vi "Periodic Tasks.vi"(8 "error in":errorcluster) -> ()   [LabVIEW 2013]
doc: "This VI runs in parallel to other tasks. It can contain as many user-defined periodic loops as you need. These can carry out PID or other sorts of timed response."
uses:
  <vilib>/Rock Robotics/SystemInterfaces/Utilities/FPGA_UtilitiesLED Source.ctl
  <vilib>/Rock Robotics/SystemInterfaces/Utilities/FPGA_UtilitiesLED State.ctl
  Robot Global Data.vi
  RefnameEnum.ctl
  SingleSolenoidAction.ctl
  TankDriveAction.ctl
  RollerAction.ctl
  DoubleSolenoidAction.ctl
panel:
  out "Collector Timer":dbl
  out "Clapper Timer":dbl
  out "Roller Pneumatic Timer":dbl
  out "Firing Cylinder Timer":dbl
  out "Sonic Shifter Timer":dbl
  out "Kicker Timer":dbl
  out "Roller Motor Timer":dbl
  out "Tank Drive Timer":dbl
  in  "LowerSpeed":dbl=-0.5
  in  "RaiseSpeed":dbl=0.5
  # "COLLECTOR ARM"
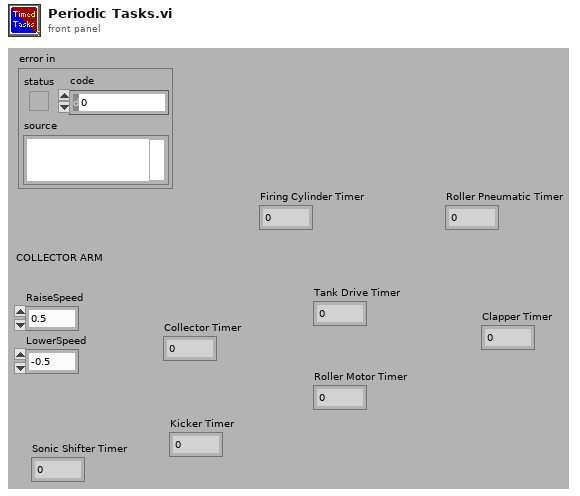
[diagram p1: front panel]
types:
  T1 = typedef "RefnameEnum.ctl" = enum16{"TankDrive", "Controller1", "Controller2", "SonicShifter", "Compressor"}
  T2 = typedef "SingleSolenoidAction.ctl" = enum16{"Init", "SetState", "Disable"}
  T3 = typedef "WPI_CompressorDevRef.ctl" = cluster{"DevStatus":errorcluster, "DigitalInputDevRef":T4, "RelayDevRef":T7}
  T4 = typedef "WPI_DigitalInputDevRef.ctl" = cluster{"DevStatus":errorcluster, "DIO Channel":T5, "Digital Module":T6}
  T5 = typedef "FPGA_DIOChannel.ctl" = enum8{"DIO 1", "DIO 2", "DIO 3", "DIO 4", "DIO 5", "DIO 6", "DIO 7", "DIO 8", "DIO 9", "DIO 10", "DIO 11", "DIO 12", "DIO 13", "DIO 14", "Invalid"}
  T6 = typedef "FPGA_TypedefDigitalModule.ctl" = enum16{"Digital Module 1", "Digital Module 2"}
  T7 = typedef "WPI_RelayDevRef.ctl" = cluster{"DevStatus":errorcluster, "Relay Channel":T8, "Digital Module":T6, "Relay Direction":T9}
  T8 = typedef "FPGA_DIORelayChannel.ctl" = enum8{"Relay 1", "Relay 2", "Relay 3", "Relay 4", "Relay 5", "Relay 6", "Relay 7", "Relay 8", "Invalid"}
  T9 = typedef "WPI_RelayDirection.ctl" = enum16{"Both directions", "Forward only", "Reverse only"}
  T10 = typedef "TankDriveAction.ctl" = enum16{"Init", "LinearDrive", "SetValue", "Disable"}
  T11 = typedef "DoubleSolenoidAction.ctl" = enum16{"Init", "Middle", "In", "Out"}
  T12 = typedef "CollectorAction.ctl" = enum16{"Init", "Raise", "Lower", "Stop", "GetStatus"}
  T13 = typedef "RollerAction.ctl" = enum16{"Init", "Off", "Forward", "Reverse"}
  T14 = typedef "FPGA_UtilitiesLED State.ctl" = enum16{"Off", "On", "Toggle"}
  T15 = typedef "FPGA_UtilitiesLED Source.ctl" = enum16{"User LED", "FPGA LED"}
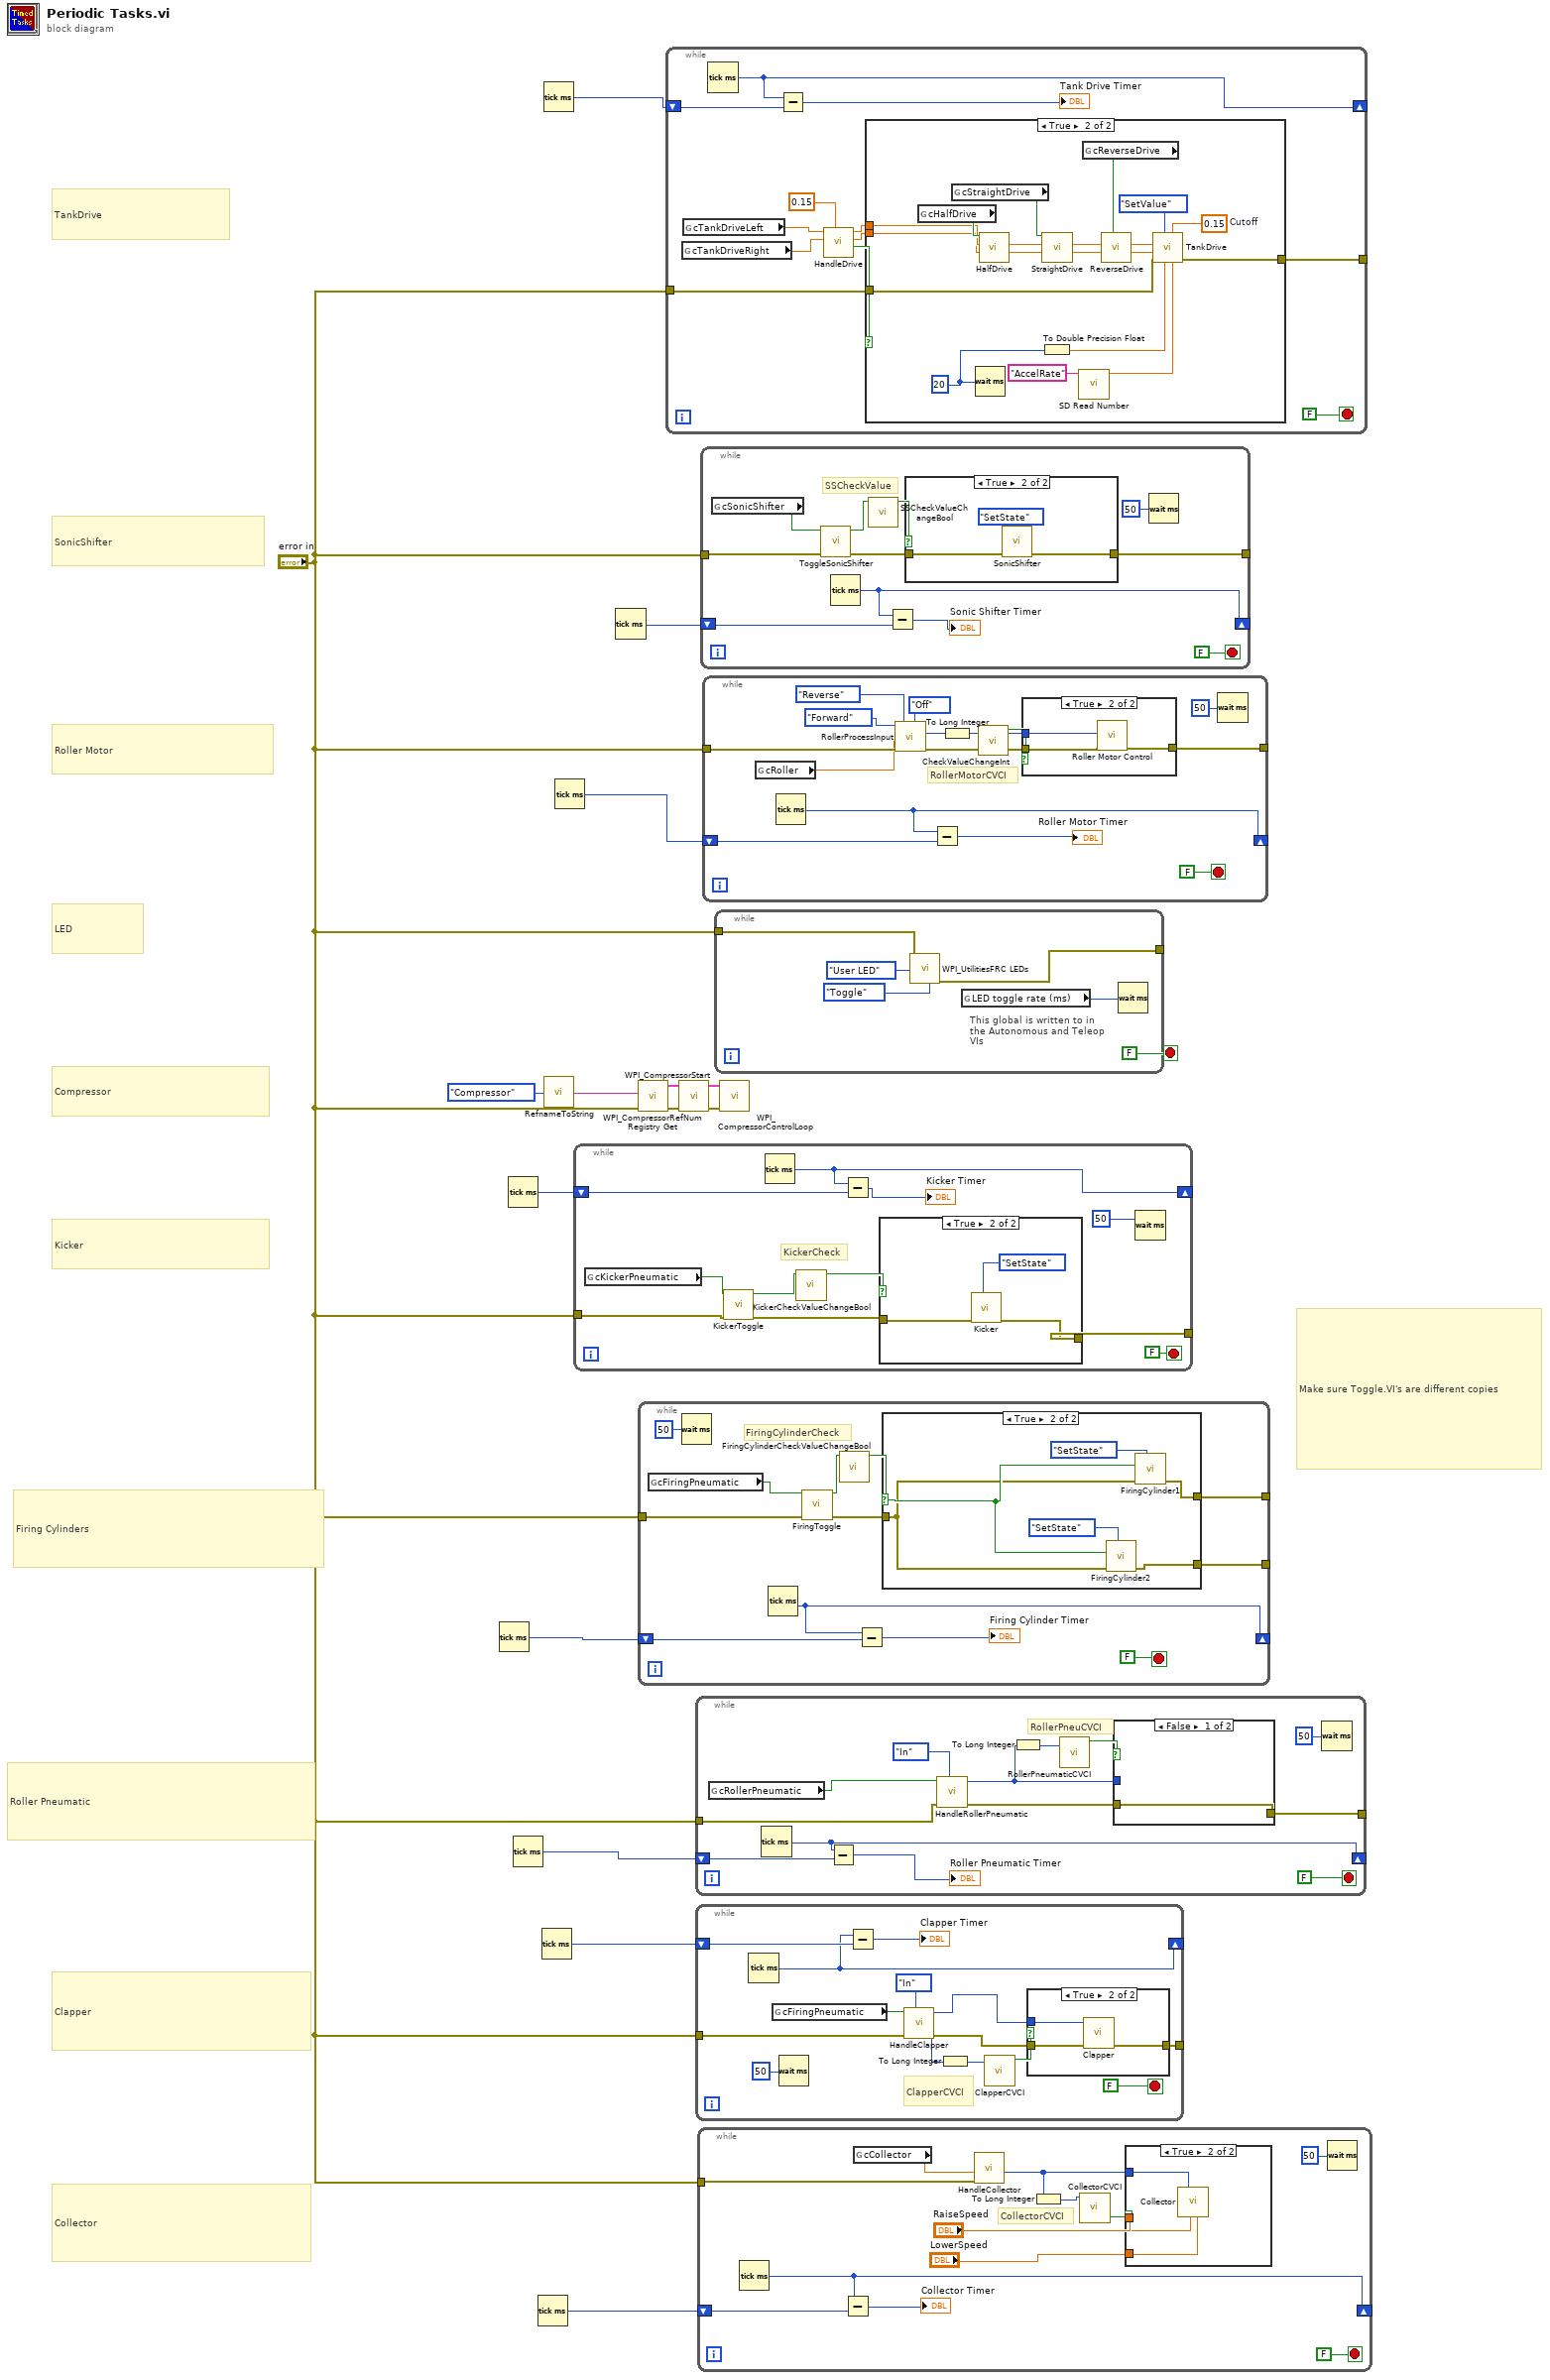
[diagram p0: block diagram]
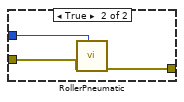
[diagram p4: hidden frame]
diagram:
  # "Collector"
  # "Clapper"
  # "Roller Pneumatic"
  # "Make sure Toggle.VI's are different copies"
  # "Firing Cylinders"
  # "Kicker"
  # "Compressor"
  # "Roller Motor"
  # "SonicShifter"
  # "LED"
  # "TankDrive"
  n1 = Tick Count (ms)() -> (millisecond timer value=w4:u32)
  n2 = Tick Count (ms)() -> (millisecond timer value=w5:u32)
  n3 = Tick Count (ms)() -> (millisecond timer value=w3:u32)
  n4 = Tick Count (ms)() -> (millisecond timer value=w6:u32)
  n5 = Tick Count (ms)() -> (millisecond timer value=w2:u32)
  n6 = Tick Count (ms)() -> (millisecond timer value=w9:u32)
  n7 = call "RefnameToString.vi"("Enum"=RefnameEnum."Compressor") -> ("Refname"=w13:string)
  n8 = Tick Count (ms)() -> (millisecond timer value=w7:u32)
  n9 = while {
    tunnel: "error in" -> [w20]
    shift-right: [w22] -> _
    shift-left: w5 -> [w24]
    tunnel: [w21] -> _
    stop <- FALSE stop-if-true
    # "KickerCheck"
    n10 = global read "Robot Global Data.vi" "cKickerPneumatic"() -> (w18:bool)
    n11 = call "KickerToggle.vi"("error in"=w20, "RawInput"=w18) -> ("error out"=w19:errorcluster, "ToggleState"=w17:bool)  [unwired: 8 in]
    n12 = Tick Count (ms)() -> (millisecond timer value=w22:u32)
    n13 = call "KickerCheckValueChangeBool.vi"("Input Boolean"=w17) -> ("Boolean Changed?"=w16:bool)  [unwired: 10 in]
    n14 = Subtract(x=w22, y=w24) -> (x-y=→"Kicker Timer":u32)
    n15 = case shown="True" w16 {
      tunnel: w19 -> [w27 w28]
      tunnel: [w27 w29] -> w21
      frame False {
      }
      frame True {
        n16 = call "Kicker.vi"("Action"=SingleSolenoidAction."SetState", "error in (no error)"=w28) -> ("error out"=w29:errorcluster)  [unwired: 9 in]
      }
    }
    n17 = Wait (ms)(milliseconds to wait=u32 50) -> ()  [unwired: 1 out]
  }
  n18 = Tick Count (ms)() -> (millisecond timer value=w8:u32)
  n19 = call <vilib>:"WPI_CompressorRefNum Registry Get.vi"("error in (no error)"="error in", "refnum name"=w13) -> ("error out"=w15:errorcluster, "CompressorDevRef"=w11:T3)  [unwired: 8 in]
  n20 = while {
    tunnel: "error in" -> [w34]
    shift-right: [w40] -> _
    shift-left: w4 -> [w39]
    tunnel: [w37] -> _
    tunnel: [w36] -> _
    stop <- FALSE stop-if-true
    # "FiringCylinderCheck"
    n21 = global read "Robot Global Data.vi" "cFiringPneumatic"() -> (w35:bool)
    n22 = Wait (ms)(milliseconds to wait=u32 50) -> ()  [unwired: 1 out]
    n23 = Tick Count (ms)() -> (millisecond timer value=w40:u32)
    n24 = call "FiringToggle.vi"("error in"=w34, "RawInput"=w35) -> ("error out"=w33:errorcluster, "ToggleState"=w32:bool)  [unwired: 8 in]
    n25 = call "FiringCylinderCheckValueChangeBool.vi"("Input Boolean"=w32) -> ("Boolean Changed?"=w31:bool)  [unwired: 10 in]
    n26 = Subtract(x=w40, y=w39) -> (x-y=→"Firing Cylinder Timer":u32)
    n27 = case shown="True" w31 {
      selector: w31 -> [_ w45]
      tunnel: w33 -> [w43 w44]
      tunnel: [w43 w47] -> w37
      tunnel: [w43 w46] -> w36
      frame False {
      }
      frame True {
        n28 = call "FiringCylinder2.vi"("Action"=SingleSolenoidAction."SetState", "error in (no error)"=w44, "Actuate?"=w45) -> ("error out"=w46:errorcluster)  [unwired: 8 in]
        n29 = call "FiringCylinder1.vi"("Action"=SingleSolenoidAction."SetState", "error in (no error)"=w44, "Actuate?"=w45) -> ("error out"=w47:errorcluster)  [unwired: 8 in]
      }
    }
  }
  n30 = while {
    tunnel: "error in" -> [w51]
    shift-right: [w60] -> _
    shift-left: w9 -> [w59]
    tunnel: [w52] -> _
    stop <- FALSE stop-if-true
    n31 = global read "Robot Global Data.vi" "cTankDriveRight"() -> (w57:dbl)
    n32 = global read "Robot Global Data.vi" "cTankDriveLeft"() -> (w56:dbl)
    n33 = Tick Count (ms)() -> (millisecond timer value=w60:u32)
    n34 = Subtract(x=w60, y=w59) -> (x-y=→"Tank Drive Timer":u32)
    n35 = call "HandleDrive.vi"("Deadzone"=0.15, "RightMotor"=w57, "LeftMotor"=w56) -> ("Enqueue?"=w55:bool, "RightMotor"=w53:dbl, "LeftMotor"=w54:dbl)  [unwired: 6 in]
    n36 = case shown="True" w55 {
      tunnel: w54 -> [_ w66]
      tunnel: w53 -> [_ w65]
      tunnel: [w62 w64] -> w52
      tunnel: w51 -> [w62 w63]
      frame False {
      }
      frame True {
        w76 = 0.15  # Cutoff
        w81 = u32 20 ("milliseconds to wait")
        n37 = global read "Robot Global Data.vi" "cHalfDrive"() -> (w73:bool)
        n38 = global read "Robot Global Data.vi" "cStraightDrive"() -> (w72:bool)
        n39 = Wait (ms)(milliseconds to wait=w81) -> ()  [unwired: 1 out]
        n40 = call "HalfDrive.vi"("RightDrive in"=w65, "LeftDrive in"=w66, "HalfDrive"=w73) -> ("RightDrive out"=w75:dbl, "LeftDrive out"=w74:dbl)  [unwired: 7 in]
        n41 = call "StraightDrive.vi"("RightDrive in"=w75, "LeftDrive in"=w74, "StraightDrive"=w72) -> ("RightDrive out"=w70:dbl, "LeftDrive out"=w71:dbl)  [unwired: 7 in]
        n42 = To Double Precision Float(number=w81) -> (double precision float=w79:dbl)
        n43 = call <vilib>:"SD Read Number.vi"("Name"="AccelRate") -> ("Numeric"=w78:dbl)  [unwired: 8 in, 2 out]
        n44 = global read "Robot Global Data.vi" "cReverseDrive"() -> (w67:bool)
        n45 = call "ReverseDrive.vi"("cReverseDrive"=w67, "Right"=w70, "Left"=w71) -> ("Right"=w68:dbl, "Left"=w69:dbl)  [unwired: 7 in]
        n46 = call "TankDrive.vi"("AccelRate"=w78, "Cutoff"=w76, "LoopTime"=w79, "DriveAction"=TankDriveAction."SetValue", "error in (no error)"=w63, "RightDesired"=w68, "LeftDesired"=w69) -> ("error out"=w64:errorcluster)  [unwired: 4 in]
      }
    }
  }
  n47 = call <vilib>:"WPI_CompressorStart.vi"("error in (no error)"=w15, "CompressorDevRef"=w11) -> ("error out"=w14:errorcluster, "CompressorDevRef"=w10:T3)  [unwired: 8 in]
  n48 = while {
    tunnel: "error in" -> [w90]
    shift-right: [w89] -> _
    shift-left: w3 -> [w88]
    tunnel: [w82] -> _
    stop <- FALSE stop-if-true
    # "RollerPneuCVCI"
    n49 = global read "Robot Global Data.vi" "cRollerPneumatic"() -> (w92:bool)
    n50 = Tick Count (ms)() -> (millisecond timer value=w89:u32)
    n51 = Subtract(x=w89, y=w88) -> (x-y=→"Roller Pneumatic Timer":u32)
    n52 = call "HandleRollerPneumatic.vi"("InitState"=DoubleSolenoidAction."In", "error in (no error)"=w90, "Toggle?"=w92) -> ("error out"=w83:errorcluster, "State"=w84:T11)  [unwired: 7 in]
    n53 = To Long Integer(number=w84) -> (32bit integer=w86:i32)
    n54 = call "RollerPneumaticCVCI.vi"("Integer"=w86) -> ("CheckValueChangeInt"=w85:bool)  [unwired: 10 in]
    n55 = case shown="False" w85 {
      tunnel: w84 -> [_ w98]
      tunnel: w83 -> [w95 w97]
      tunnel: [w95 w96] -> w82
      frame False {
      }
      frame True {
        n56 = call "RollerPneumatic.vi"("State"=w98, "Error in"=w97) -> ("Error out"=w96:errorcluster)  [unwired: 9 in]
      }
    }
    n57 = Wait (ms)(milliseconds to wait=u32 50) -> ()  [unwired: 1 out]
  }
  n58 = while {
    tunnel: "error in" -> [w107]
    shift-right: [w104] -> _
    shift-left: w2 -> [w106]
    tunnel: [w101] -> _
    stop <- FALSE stop-if-true
    # "ClapperCVCI"
    n59 = Tick Count (ms)() -> (millisecond timer value=w104:u32)
    n60 = global read "Robot Global Data.vi" "cFiringPneumatic"() -> (w109:bool)
    n61 = Wait (ms)(milliseconds to wait=u32 50) -> ()  [unwired: 1 out]
    n62 = Subtract(x=w104, y=w106) -> (x-y=→"Clapper Timer":u32)
    n63 = call "HandleClapper.vi"("InitState"=DoubleSolenoidAction."In", "error in (no error)"=w107, "Toggle?"=w109) -> ("error out"=w102:errorcluster, "State"=w99:T11)  [unwired: 7 in]
    n64 = To Long Integer(number=w99) -> (32bit integer=w100:i32)
    n65 = call "ClapperCVCI.vi"("Integer"=w100) -> ("CheckValueChangeInt"=w103:bool)  [unwired: 10 in]
    n66 = case shown="True" w103 {
      tunnel: w99 -> [_ w115]
      tunnel: w102 -> [w112 w114]
      tunnel: [w112 w113] -> w101
      frame False {
      }
      frame True {
        n67 = call "Clapper.vi"("State"=w115, "Error in"=w114) -> ("Error out"=w113:errorcluster)  [unwired: 9 in]
      }
    }
  }
  n68 = while {
    tunnel: "error in" -> [w125]
    shift-right: [w122] -> _
    shift-left: w6 -> [w123]
    stop <- FALSE stop-if-true
    # "CollectorCVCI"
    n69 = Tick Count (ms)() -> (millisecond timer value=w122:u32)
    n70 = Subtract(x=w122, y=w123) -> (x-y=→"Collector Timer":u32)
    n71 = global read "Robot Global Data.vi" "cCollector"() -> (w126:dbl)
    n72 = call "HandleCollector.vi"("error in"=w125, "JoystickValue"=w126) -> ("CollectorEnum Input"=w116:T12)  [unwired: 8 in, 1 out]
    n73 = To Long Integer(number=w116) -> (32bit integer=w120:i32)
    n74 = call "CollectorCVCI.vi"("Integer"=w120) -> ("CheckValueChangeInt"=w119:bool)  [unwired: 10 in]
    n75 = case shown="True" w119 {
      tunnel: "RaiseSpeed" -> [_ w130]
      tunnel: "LowerSpeed" -> [_ w129]
      tunnel: w116 -> [_ w128]
      frame False {
      }
      frame True {
        n76 = call "Collector.vi"("LowerSpeed"=w129, "RaiseSpeed"=w130, "Action"=w128) -> ()  [unwired: 6 in, 3 out]
      }
    }
    n77 = Wait (ms)(milliseconds to wait=u32 50) -> ()  [unwired: 1 out]
  }
  n78 = while {
    tunnel: "error in" -> [w134]
    shift-right: [w138] -> _
    shift-left: w8 -> [w139]
    tunnel: [w136] -> _
    stop <- FALSE stop-if-true
    # "SSCheckValue"
    n79 = global read "Robot Global Data.vi" "cSonicShifter"() -> (w135:bool)
    n80 = call "ToggleSonicShifter.vi"("error in"=w134, "cSonicShifter"=w135) -> ("error out"=w133:errorcluster, "Actuate?"=w132:bool)  [unwired: 8 in]
    n81 = Tick Count (ms)() -> (millisecond timer value=w138:u32)
    n82 = call "SSCheckValueChangeBool.vi"("Input Boolean"=w132) -> ("Boolean Changed?"=w131:bool)  [unwired: 10 in]
    n83 = Subtract(x=w138, y=w139) -> (x-y=→"Sonic Shifter Timer":u32)
    n84 = case shown="True" w131 {
      tunnel: [w142 w144] -> w136
      tunnel: w133 -> [w142 w143]
      frame False {
      }
      frame True {
        n85 = call "SonicShifter.vi"("Action"=SingleSolenoidAction."SetState" ("Mode"), "error in (no error)"=w143) -> ("error out"=w144:errorcluster)  [unwired: 9 in]
      }
    }
    n86 = Wait (ms)(milliseconds to wait=u32 50) -> ()  [unwired: 1 out]
  }
  n87 = while {
    tunnel: "error in" -> [w155]
    shift-right: [w153] -> _
    shift-left: w7 -> [w151]
    tunnel: [w146] -> _
    stop <- FALSE stop-if-true
    # "RollerMotorCVCI"
    n88 = global read "Robot Global Data.vi" "cRoller"() -> (w154:dbl)
    n89 = Tick Count (ms)() -> (millisecond timer value=w153:u32)
    n90 = call "RollerProcessInput.vi"("OffState"=RollerAction."Off", "ReverseState"=RollerAction."Reverse", "error in"=w155, "JoystickValue"=w154, "ForwardState"=RollerAction."Forward") -> ("error out"=w147:errorcluster, "StateOut"=w148:T13)  [unwired: 5 in]
    n91 = Subtract(x=w153, y=w151) -> (x-y=→"Roller Motor Timer":u32)
    n92 = To Long Integer(number=w148) -> (32bit integer=w150:i32)
    n93 = call "CheckValueChangeInt.vi"("Integer"=w150) -> ("CheckValueChangeInt"=w149:bool)  [unwired: 10 in]
    n94 = case shown="True" w149 {
      tunnel: w148 -> [_ w164]
      tunnel: w147 -> [w161 w163]
      tunnel: [w161 w162] -> w146
      frame False {
      }
      frame True {
        n95 = call "Roller Motor Control.vi"("Action"=w164, "Error in"=w163) -> ("Error out"=w162:errorcluster)  [unwired: 9 in]
      }
    }
    n96 = Wait (ms)(milliseconds to wait=u32 50) -> ()  [unwired: 1 out]
  }
  n97 = while {
    tunnel: "error in" -> [w166]
    tunnel: [w165] -> _
    stop <- FALSE stop-if-true
    # "This global is written to in the Autonomous and Teleop VIs"
    n98 = call <vilib>:"WPI_UtilitiesFRC LEDs.vi"("error in (no error)"=w166, "State"=FPGA_UtilitiesLED_State."Toggle", "LED Type"=FPGA_UtilitiesLED_Source."User LED") -> ("error out"=w165:errorcluster)  [unwired: 8 out]
    n99 = global read "Robot Global Data.vi" "LED toggle rate (ms)"() -> (w167:u32)
    n100 = Wait (ms)(milliseconds to wait=w167) -> ()  [unwired: 1 out]
  }
  n101 = call <vilib>:"WPI_CompressorControlLoop.vi"("error in (no error)"=w14, "CompressorDevRef"=w10) -> ()  [unwired: 10 in]
